vi "Instr get_param_type.vi"(1 "value_array":string) -> (0 "type":string)   [LabVIEW 2018]
uses:
  <vilib>/regexp/Match Regular Expression.xnode
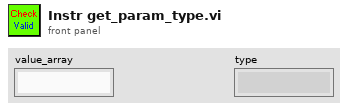
[diagram p1: front panel]
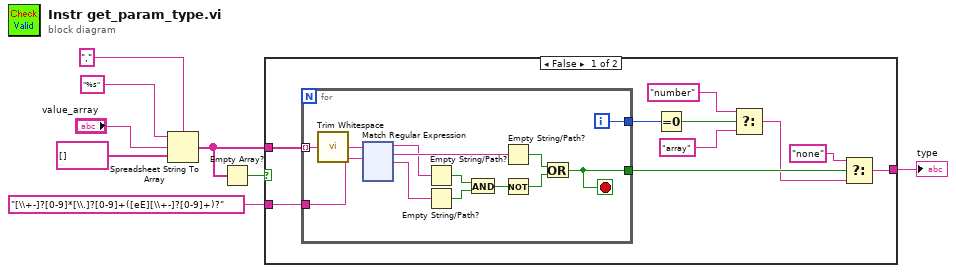
[diagram p0: block diagram]
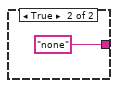
[diagram p2: hidden frame]
diagram:
  n1 = Spreadsheet String To Array(delimiter (Tab)=",", format string="%s", spreadsheet string="value_array", array type (2D Dbl)=string[] []) -> (array=w4:string[])
  n2 = Empty Array?(array=w4) -> (empty?=w3:bool)
  n3 = case shown="False" w3 {
    tunnel: "[\\+-]?[0-9]*[\\.]?[0-9]+([eE][\\+-]?[0-9]+)?" ("regular expression") -> [w18 _]
    tunnel: w4 -> [w17 _]
    tunnel: [w9 "none"] -> w2
    frame False {
      n4 = for {
        tunnel: w18 -> [w31]
        tunnel: w17 -> [w28] mode=indexing
        tunnel: [w19] -> w14
        tunnel: [w29] -> w16
        i -> [w29]
        stop <- w19 stop-if-true
        n5 = call <vilib>:"Trim Whitespace.vi"("string"=w28) -> ("trimmed string"=w27:string)  [unwired: 1 in]
        n6 = xnode "Match Regular Expression"("input string"=w27, "regular expression"=w31) -> ("before match"=w26:string, "whole match"=w30:string, "after match"=w25:string)  [unwired: 4 in, 2 out]
        n7 = Empty String/Path?(string/path=w26) -> (empty?=w24:bool)
        n8 = Empty String/Path?(string/path=w25) -> (empty?=w23:bool)
        n9 = And(x=w24, y=w23) -> (x .and. y?=w22:bool)
        n10 = Empty String/Path?(string/path=w30) -> (empty?=w21:bool)
        n11 = Not(x=w22) -> (.not. x?=w20:bool)
        n12 = Or(x=w21, y=w20) -> (x .or. y?=w19:bool)
      }
      n13 = Equal To 0?(x=w16) -> (x = 0?=w15:bool)
      n14 = Select(t="number", s=w15, f="array") -> (s? t:f=w10:string)
      n15 = Select(t="none", s=w14, f=w10) -> (s? t:f=w9:string)
    }
    frame True {
    }
  }
  "type" <- w2
